vi "消除.vi"(11 "数组":u32[][](array[colorbox])) -> (2 "得分":i8, 3 "数组 2":u32[][](array[colorbox]))   [LabVIEW 2012]
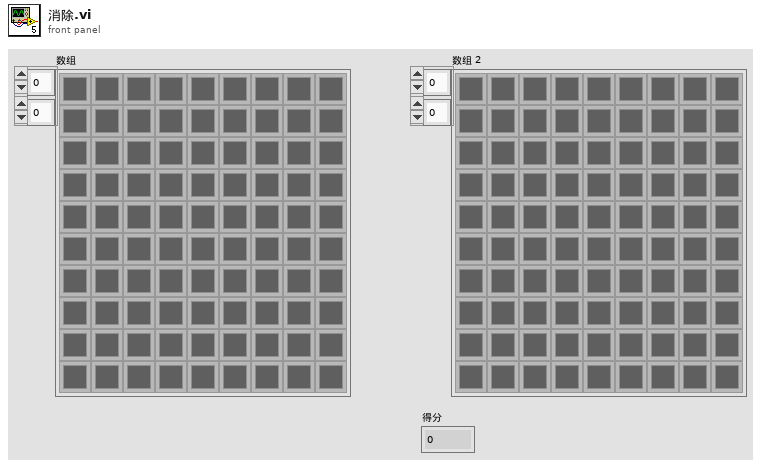
[diagram p1: front panel]
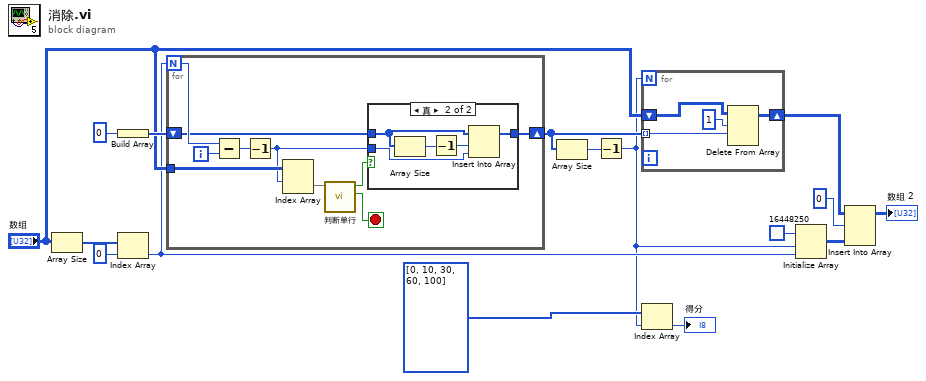
[diagram p0: block diagram]
diagram:
  n1 = Array Size(array="数组") -> (size(s)=w16:i32[])
  n2 = Build Array(0) -> (w13:i32[])
  n3 = Index Array(array=w16, index=0 ("索引")) -> (element=w8:i32)
  n4 = for {
    N: w8 -> [w26]
    tunnel: "数组" -> [w24]
    shift-right: [w19] -> w11
    shift-left: w13 -> [w21]
    i -> [w20]
    stop <- w23 stop-if-true
    n5 = Subtract(x=w26, y=w20) -> (x-y=w18:i32)
    n6 = Decrement(x=w18) -> (x-1=w17:i32)
    n7 = Index Array(array=w24, index (row)=w17) -> (element=w25:u32[])  [unwired: 1 in]
    n8 = call "判断单行.vi"("数组"=w25) -> ("是否空行"=w23:bool, "是否满行"=w22:bool)  [unwired: 9 in]
    n9 = case shown="真" w22 {
      tunnel: w21 -> [w27 w30]
      tunnel: w17 -> [_ w31]
      tunnel: [w27 w32] -> w19
      frame False {
      }
      frame True {
        n10 = Array Size(array=w30) -> (size(s)=w29:i32)
        n11 = Decrement(x=w29) -> (x-1=w28:i32)
        n12 = Insert Into Array(array=w30, index=w28, new element=w31) -> (w32:i32[])
      }
    }
  }
  n13 = Array Size(array=w11) -> (size(s)=w4:i32)
  n14 = Decrement(x=w4) -> (x-1=w1:i32)
  n15 = for {
    N: w1 -> [_]
    tunnel: w11 -> [w34] mode=indexing
    shift-right: [w35] -> w10
    shift-left: "数组" -> [w36]
    n16 = Delete From Array(array=w36, length=1 ("长度"), index (row)=w34) -> (array with subset deleted=w35:u32[][])  [unwired: 1 in, 1 out]
  }
  n17 = Index Array(array=i32[] [0, 10, 30, 60, 100], index=w1) -> (element=→"得分":i32)
  n18 = Initialize Array(u32 16448250, w1, w8) -> (w6:u32[][])
  n19 = Insert Into Array(array=w10, index (row)=0 ("索引 (行)"), new element=w6) -> (→"数组 2":u32[][])  [unwired: 1 in]
